vi "RT Main.vi"() -> ()   [LabVIEW 2017]
doc: "Demonstrates the use of the UDP functions to receive broadcast data over a UDP connection."
uses:
  <vilib>/myRIO/Instrument Drivers/Utilities/Utilities.lvlib
panel:
  out "error out":errorcluster
  in  "Stop":bool
  # "Overview: Demonstrates the use of the UDP functions to receive broadcast data over a UDP connection.\nInstructions:\n1. Ensure Desktop Main.vi is already running.\n2. Run this VI.\n3. After you change the value of LED on Desktop Main.vi, observe the value change of LED Status on this VI.\n4. Click Stop to stop this VI."
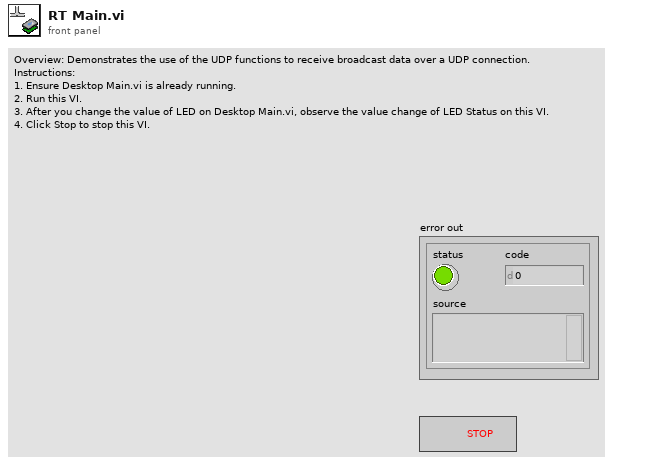
[diagram p1: front panel]
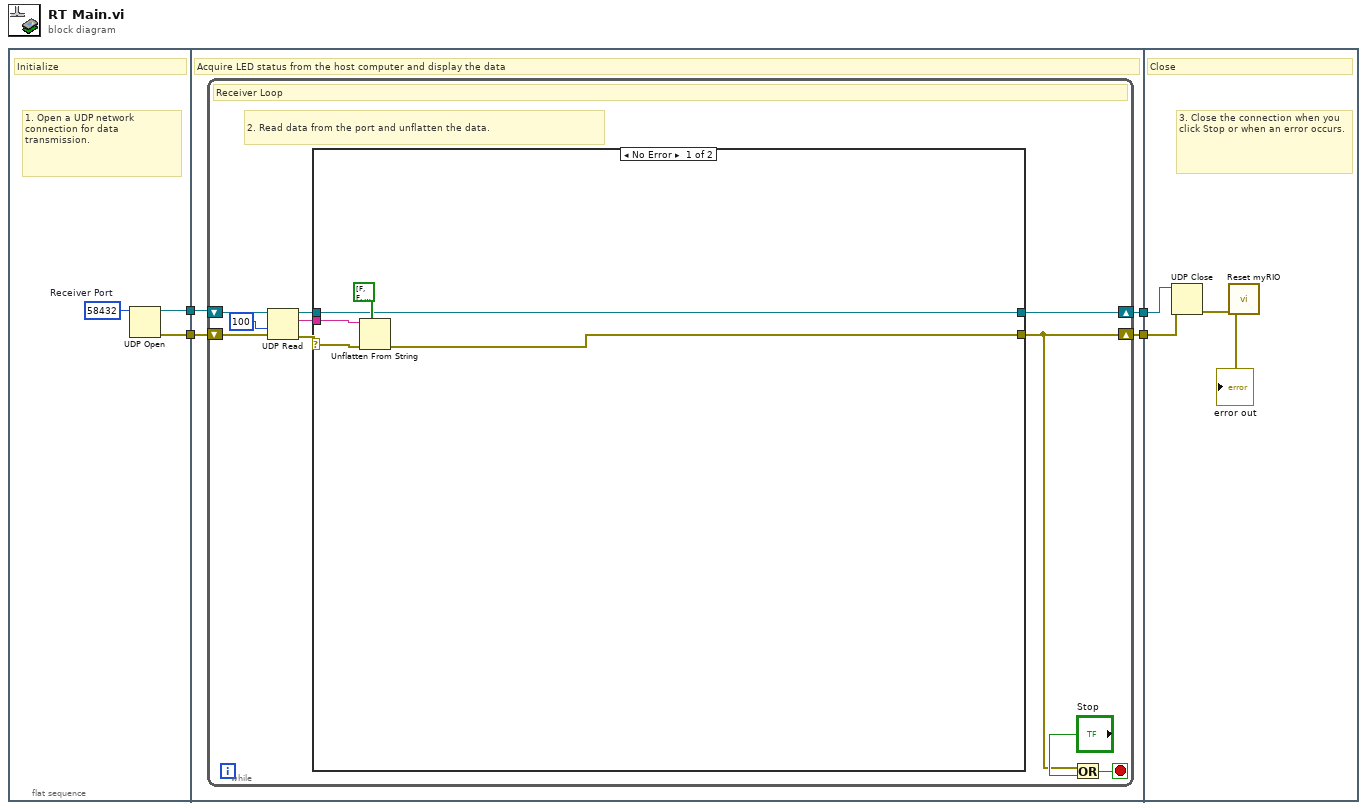
[diagram p0: block diagram]
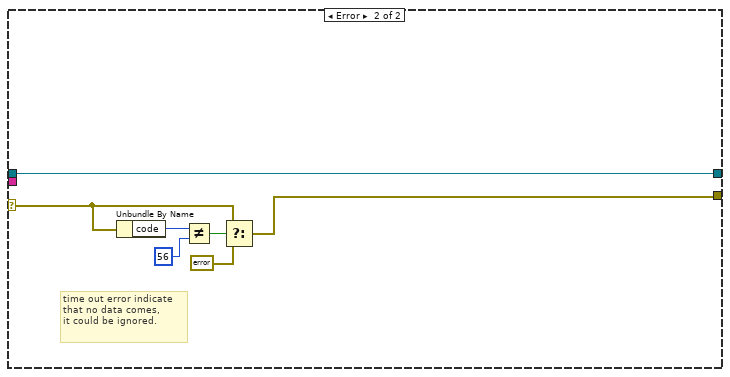
[diagram p2: hidden frame]
diagram:
  n1 = flat-sequence {
    tunnel: [w6] -> w2
    tunnel: [w5] -> w1
    tunnel: [w11] -> w4
    tunnel: [w10] -> w3
    tunnel: w2 -> [w9]
    tunnel: w1 -> [w8]
    tunnel: w4 -> [w37]
    tunnel: w3 -> [w38]
    frame #0 {
      w7 = u16 58432  # Receiver Port
      # "1. Open a UDP network connection for data transmission."
      # "Initialize"
      n2 = UDP Open(11:w7) -> (port=w6:refnum<k16>, 0:w5:errorcluster)  [unwired: 4 in, 1 out]
    }
    frame #1 {
      # "Acquire LED status from the host computer and display the data"
      n3 = while {
        shift-right: [w14] -> w10
        shift-left: w8 -> [w20]
        shift-right: [w12] -> w11
        shift-left: w9 -> [w21]
        stop <- w16 stop-if-true
        # "2. Read data from the port and unflatten the data."
        # "Receiver Loop"
        n4 = UDP Read(connection ID=w21, timeout ms (25000)=100, 8:w20) -> (data out=w19:string, error out=w15:errorcluster, 3:w13:refnum<k16>)  [unwired: 1 in, 2 out]
        n5 = case shown="No Error" w15 {
          selector: w15 -> [w26 w29]
          tunnel: [w22 w28] -> w14
          tunnel: w19 -> [w27 _]
          tunnel: w13 -> [w23 w34]
          tunnel: [w23 w34] -> w12
          frame No Error {
            n6 = Unflatten From String(type=bool[] [FALSE, FALSE, FALSE, FALSE] ("LED Status"), binary string=w27, error in (no error)=w26) -> (value=w24:bool[], error out=w22:errorcluster)  [unwired: 2 in, 1 out]
          }
          frame Error {
            # "time out error indicate that no data comes,\nit could be ignored."
            n7 = Unbundle By Name(w29) -> ("code"=w31:i32)
            n8 = Not Equal?(x=w31, y=56) -> (x != y?=w30:bool)
            n9 = Select(t=w29, s=w30, f=errorcluster {"status"=FALSE, "code"=0, "source"=""} ("error out")) -> (s? t:f=w28:errorcluster)
          }
        }
        n10 = Or(x=w14, y="Stop") -> (x .or. y?=w16:bool)
      }
    }
    frame #2 {
      # "3. Close the connection when you click Stop or when an error occurs."
      # "Close"
      n11 = UDP Close(connection ID=w37, 8:w38) -> (error out=w36:errorcluster)  [unwired: 1 out]
      n12 = call <vilib>:"Reset myRIO.vi"("error in (no error)"=w36) -> ("error out"=→"error out":errorcluster)  [unwired: 10 in]
    }
  }
